vi "SetComponent.vi"(0 "reference in":refnum<class "MES_Base.lvclass">, 5 "Name":string, 7 "SN":string, 9 "BN":string, 11 "error in (no error)":errorcluster) -> (4 "reference in":refnum<class "MES_Base.lvclass">, 15 "error out":errorcluster)   [LabVIEW 2022 SP3, in "MES_Base.lvlib" / "MES_Base.lvclass"]
uses:
  MES_Base.lvclass
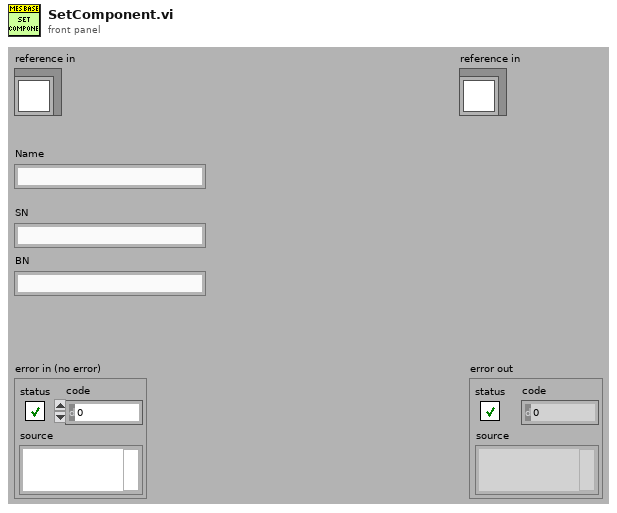
[diagram p1: front panel]
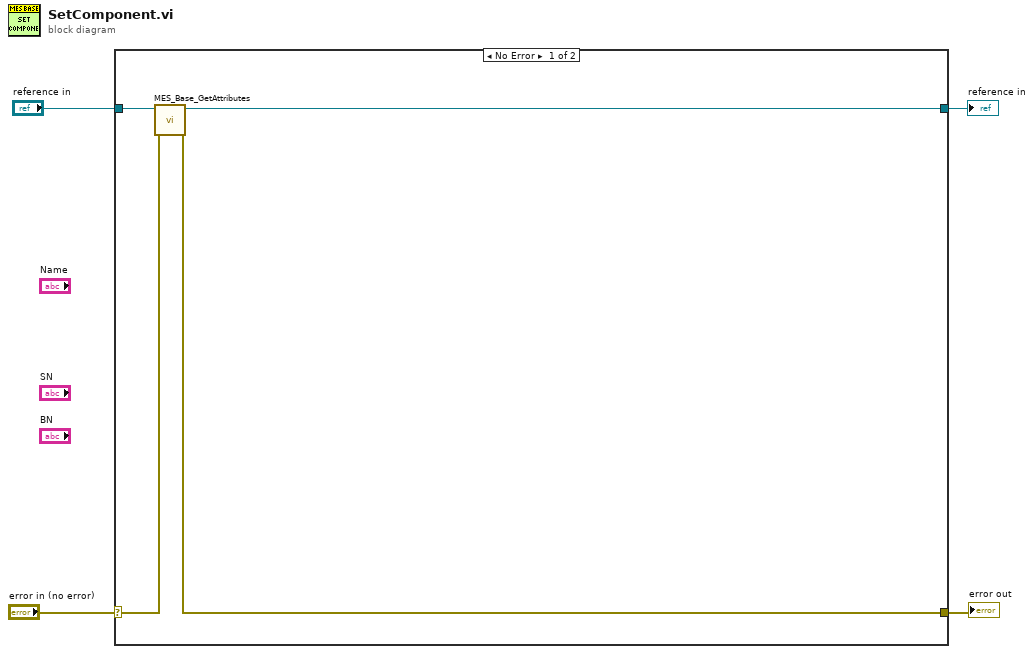
[diagram p0: block diagram]
diagram:
  n1 = case shown="No Error" "error in (no error)" {
    selector: "error in (no error)" -> [w8 w10]
    tunnel: [w5 w10] -> w3
    tunnel: [w6 w9] -> w1
    tunnel: "reference in" -> [w7 w9]
    frame No Error {
      n2 = call "MES_Base_GetAttributes.vi"("error in (no error)"=w8, "reference in"=w7) -> ("error out"=w5:errorcluster, "reference out"=w6:refnum<class "MES_Base.lvclass">)  [unwired: 6 in, 2 out]
    }
    frame Error {
    }
  }
  "error out" <- w3
  "reference in" <- w1
